vi "init.vi"() -> ()   [LabVIEW 2024]
uses:
  globalVar.vi
panel:
  in  "ring":u16[][](array[ring])
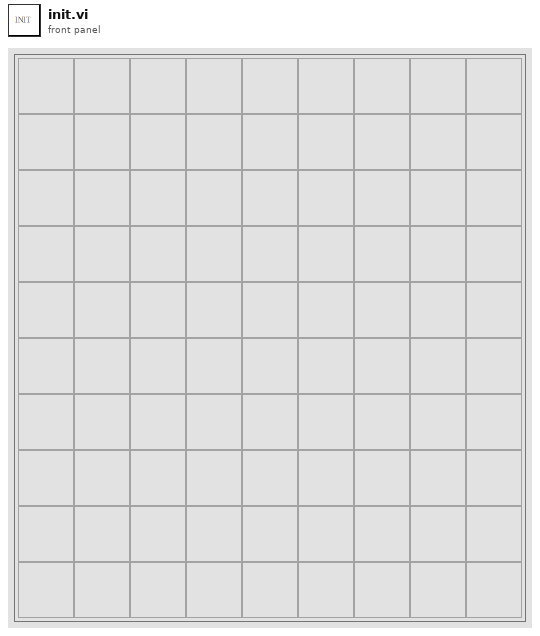
[diagram p1: front panel]
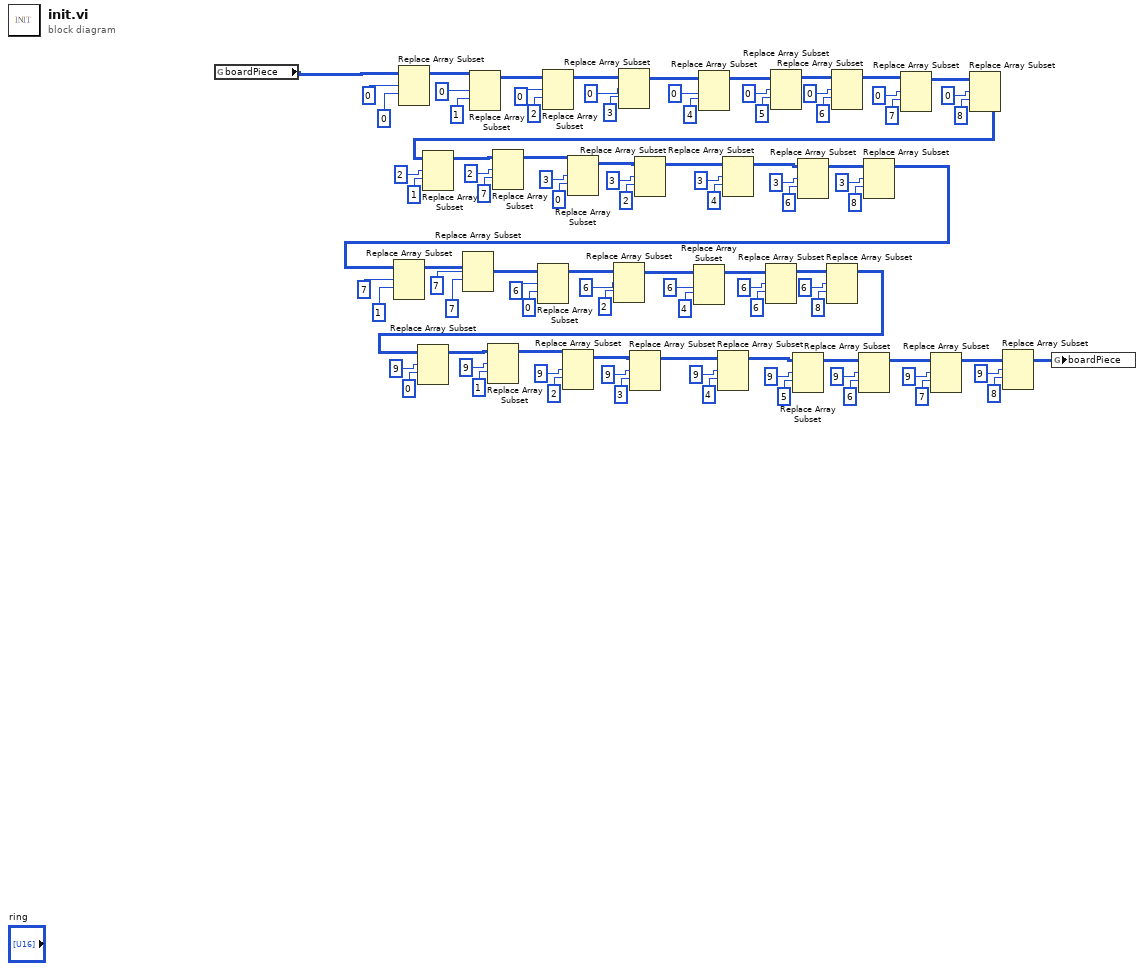
[diagram p0: block diagram]
diagram:
  n1 = global read "globalVar.vi" "boardPiece"() -> (w2:i32[][])
  n2 = Replace Array Subset(array=w2, index (row)=0, index (col)=0) -> (w28:i32[][])  [unwired: 1 in]
  n3 = Replace Array Subset(array=w28, index (row)=0, index (col)=1) -> (w7:i32[][])  [unwired: 1 in]
  n4 = Replace Array Subset(array=w7, index (row)=0, index (col)=2) -> (w9:i32[][])  [unwired: 1 in]
  n5 = Replace Array Subset(array=w9, index (row)=0, index (col)=3) -> (w11:i32[][])  [unwired: 1 in]
  n6 = Replace Array Subset(array=w11, index (row)=0, index (col)=4) -> (w15:i32[][])  [unwired: 1 in]
  n7 = Replace Array Subset(array=w15, index (row)=0, index (col)=5) -> (w19:i32[][])  [unwired: 1 in]
  n8 = Replace Array Subset(array=w19, index (row)=0, index (col)=6) -> (w24:i32[][])  [unwired: 1 in]
  n9 = Replace Array Subset(array=w24, index (row)=0, index (col)=7) -> (w25:i32[][])  [unwired: 1 in]
  n10 = Replace Array Subset(array=w25, index (row)=0, index (col)=8) -> (w33:i32[][])  [unwired: 1 in]
  n11 = Replace Array Subset(array=w33, index (row)=2, index (col)=1) -> (w34:i32[][])  [unwired: 1 in]
  n12 = Replace Array Subset(array=w34, index (row)=2, index (col)=7) -> (w45:i32[][])  [unwired: 1 in]
  n13 = Replace Array Subset(array=w45, index (row)=3, index (col)=0) -> (w46:i32[][])  [unwired: 1 in]
  n14 = Replace Array Subset(array=w46, index (row)=3, index (col)=2) -> (w47:i32[][])  [unwired: 1 in]
  n15 = Replace Array Subset(array=w47, index (row)=3, index (col)=4) -> (w48:i32[][])  [unwired: 1 in]
  n16 = Replace Array Subset(array=w48, index (row)=3, index (col)=6) -> (w49:i32[][])  [unwired: 1 in]
  n17 = Replace Array Subset(array=w49, index (row)=3, index (col)=8) -> (w89:i32[][])  [unwired: 1 in]
  n18 = Replace Array Subset(array=w89, index (row)=7, index (col)=1) -> (w70:i32[][])  [unwired: 1 in]
  n19 = Replace Array Subset(array=w70, index (row)=7, index (col)=7) -> (w84:i32[][])  [unwired: 1 in]
  n20 = Replace Array Subset(array=w84, index (row)=6, index (col)=0) -> (w82:i32[][])  [unwired: 1 in]
  n21 = Replace Array Subset(array=w82, index (row)=6, index (col)=2) -> (w80:i32[][])  [unwired: 1 in]
  n22 = Replace Array Subset(array=w80, index (row)=6, index (col)=4) -> (w76:i32[][])  [unwired: 1 in]
  n23 = Replace Array Subset(array=w76, index (row)=6, index (col)=6) -> (w72:i32[][])  [unwired: 1 in]
  n24 = Replace Array Subset(array=w72, index (row)=6, index (col)=8) -> (w91:i32[][])  [unwired: 1 in]
  n25 = Replace Array Subset(array=w91, index (row)=9, index (col)=0) -> (w65:i32[][])  [unwired: 1 in]
  n26 = Replace Array Subset(array=w65, index (row)=9, index (col)=1) -> (w54:i32[][])  [unwired: 1 in]
  n27 = Replace Array Subset(array=w54, index (row)=9, index (col)=2) -> (w53:i32[][])  [unwired: 1 in]
  n28 = Replace Array Subset(array=w53, index (row)=9, index (col)=3) -> (w52:i32[][])  [unwired: 1 in]
  n29 = Replace Array Subset(array=w52, index (row)=9, index (col)=4) -> (w51:i32[][])  [unwired: 1 in]
  n30 = Replace Array Subset(array=w51, index (row)=9, index (col)=5) -> (w50:i32[][])  [unwired: 1 in]
  n31 = Replace Array Subset(array=w50, index (row)=9, index (col)=6) -> (w96:i32[][])  [unwired: 1 in]
  n32 = Replace Array Subset(array=w96, index (row)=9, index (col)=7) -> (w97:i32[][])  [unwired: 1 in]
  n33 = Replace Array Subset(array=w97, index (row)=9, index (col)=8) -> (w1:i32[][])  [unwired: 1 in]
  n34 = global write "globalVar.vi" "boardPiece"(w1) -> ()
